vi "Set Device Parameter.vi"(6 "Parameter":string, 8 "error in (no error)":errorcluster, 9 "Parameter Name":string, 10 "IED Name":string, 11 "SCADA in":refnum<class "SCADA.lvclass">) -> (0 "error out":errorcluster, 3 "SCADA out":refnum<class "SCADA.lvclass">)   [LabVIEW 2015, in "SCADA Core.lvlib" / "SCADA.lvclass"]
uses:
  SCADA.lvclass
  Controls/Queue Selector.ctl
  Controls/Parameter Type.ctl
  IED Actor/IED Messages/Set Parameter Msg/Set Parameter Msg.lvclass/Set Parameter Msg.ctl
  <vilib>/ActorFramework/Message Enqueuer/Message Enqueuer.lvclass/Message Enqueuer.ctl
  SCADA Abstract Messages/Set Device Parameter Status Msg/Set Device Parameter Status.ctl
  <vilib>/ActorFramework/Actor/Actor.lvclass/Actor.ctl
  SCADA Response Messages/Return Parameter Status Msg/Return Parameter Status Msg.lvclass/Return Parameter Status Msg.ctl
  <vilib>/ActorFramework/Message Enqueuer/Enqueue.vi
  <vilib>/ActorFramework/Message Enqueuer/Init from Existing Queue.vi
  <vilib>/ActorFramework/Message Priority Queue/Priority Enqueue.vi
  IED Actor/IED Messages/Set Parameter Msg/Set Parameter Msg.lvclass
  <vilib>/ActorFramework/Message Enqueuer/Message Enqueuer.lvclass
  SCADA Response Messages/Return Parameter Status Msg/Return Parameter Status Msg.lvclass
  Utilities/Message Strings.llb/Message String Utilities.lvlib
  <vilib>/ActorFramework/Actor/Actor.lvclass
  SCADA Abstract Messages/Set Device Parameter Status Msg/Set Device Parameter Status Msg.lvclass
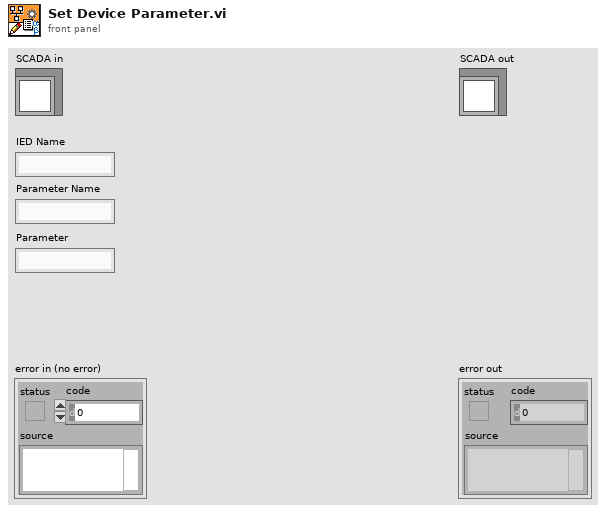
[diagram p1: front panel]
types:
  T1 = typedef "SCADA Core.lvlib/SCADA.lvclass/Parameter Type.ctl" = enum8{"Boolean", "U16", "U32", "I32", "Double", "String"}
  T2 = typedef "SCADA Core.lvlib/SCADA.lvclass/Queue Selector.ctl" = enum16{"IEDs", "PV", "Generators", "Wind", "Storage", "Relays"}
  T3 = typedef "SCADA Core.lvlib/Set Device Parameter Status Msg.lvclass/Set Device Parameter Status.ctl" = enum16{"Success", "Failure"}
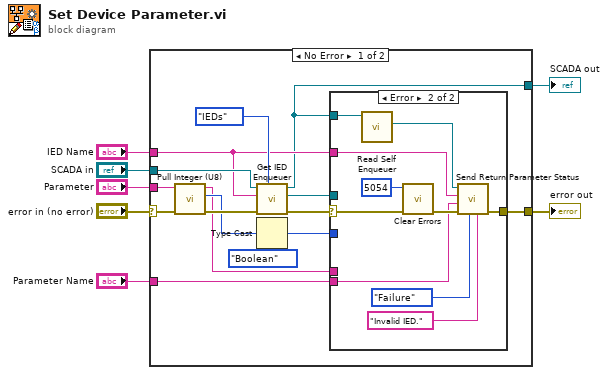
[diagram p0: block diagram]
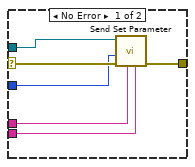
[diagram p2: hidden frame]
diagram:
  n1 = case shown="No Error" "error in (no error)" {
    selector: "error in (no error)" -> [w20 w40]
    tunnel: [w9 w40] -> w6
    tunnel: [w8 w39] -> w4
    tunnel: "SCADA in" -> [w21 w39]
    tunnel: "IED Name" -> [w14 _]
    tunnel: "Parameter Name" -> [w13 _]
    tunnel: "Parameter" -> [w18 _]
    frame No Error {
      n2 = call "Pull Integer (U8).vi"("error in (no error)"=w20, "String in"=w18) -> ("error out"=w19:errorcluster, "Integer out"=w17:u8, "Remaining String"=w10:string)  [unwired: 7 in]
      n3 = call "Get IED Enqueuer.vi"("Queue (IEDs)"=Queue_Selector."IEDs" ("Queue"), "error in (no error)"=w19, "IED Name"=w14, "SCADA in"=w21) -> ("error out"=w15:errorcluster, "IED Enqueuer"=w12:refnum<class "Message Enqueuer.lvclass">, "SCADA out"=w8:refnum<class "SCADA.lvclass">)  [unwired: 5 in]
      n4 = Type Cast(type=Parameter_Type."Boolean" ("Type"), x=w17) -> (*(type *) &x=w11:T1)
      n5 = case shown="Error" w15 {
        selector: w15 -> [w28 w37]
        tunnel: w12 -> [w26 _]
        tunnel: [w27 w34] -> w9
        tunnel: w8 -> [_ w38]
        tunnel: w14 -> [_ w31]
        tunnel: w13 -> [w23 w29]
        tunnel: w11 -> [w25 _]
        tunnel: w10 -> [w24 _]
        frame No Error {
          n6 = call "Send Set Parameter.vi"("Name"=w23, "Value"=w24, "error in (no error)"=w28, "Type"=w25, "Message Enqueuer"=w26) -> ("error out"=w27:errorcluster)  [unwired: 5 in, 1 out]
        }
        frame Error {
          n7 = call <vilib>:"Read Self Enqueuer.vi"("Actor"=w38) -> ("Self Enqueuer"=w30:refnum<class "Message Enqueuer.lvclass">)  [unwired: 10 in]
          n8 = call <vilib>:"Clear Errors.vi"("error in (no error)"=w37, "specific error code to clear (0: all)"=5054) -> ("error out"=w35:errorcluster)  [unwired: 4 in, 1 out]
          n9 = call "Send Return Parameter Status.vi"("error"="Invalid IED." ("error string"), "Status"=Set_Device_Parameter_Status."Failure", "error in (no error)"=w35, "Parameter Name"=w29, "IED Name"=w31, "Message Enqueuer"=w30) -> ("error out"=w34:errorcluster)  [unwired: 4 in, 1 out]
        }
      }
    }
    frame Error {
    }
  }
  "error out" <- w6
  "SCADA out" <- w4
